vi "getGroupIdxAndLeng.vi"(8 "error in (no error)":errorcluster, 10 "DOF Group":T1, 11 "OptStateEsti in":refnum<class "OptStateEsti.lvclass">) -> (0 "error out":errorcluster, 1 "Group Length":i32, 2 "Start Index":i32, 3 "OptStateEsti out":refnum<class "OptStateEsti.lvclass">)   [LabVIEW 2016, in "OfcFunc.lvlib" / "OptStateEsti.lvclass"]
doc: "Get the start index and length of specific group of degree of freedom (DOF)."
uses:
  OptStateEsti.lvclass
  StrictDef/DofGroup.ctl
  OptStateEsti.lvclass/OptStateEsti.ctl
  <vilib>/regexp/Match Regular Expression.xnode
  MatOper/MatOper.lvclass
  OfcFunc.lvlib
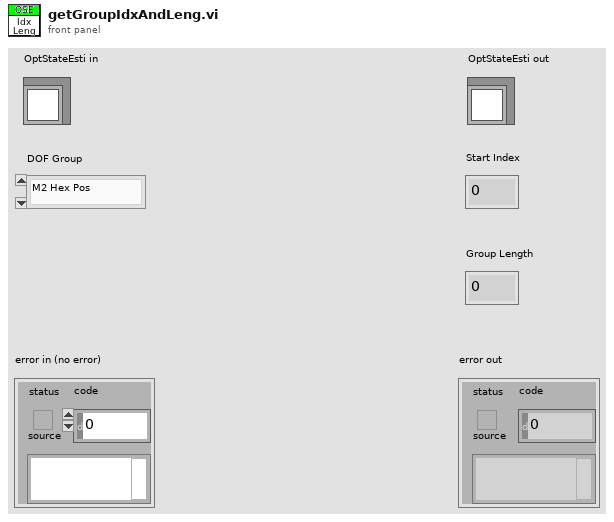
[diagram p1: front panel]
types:
  T1 = typedef "OfcFunc.lvlib/DofGroup.ctl" = enum16{"M2 Hex Pos", "Cam Hex Pos", "M1M3 Bend", "M2 Bend"}
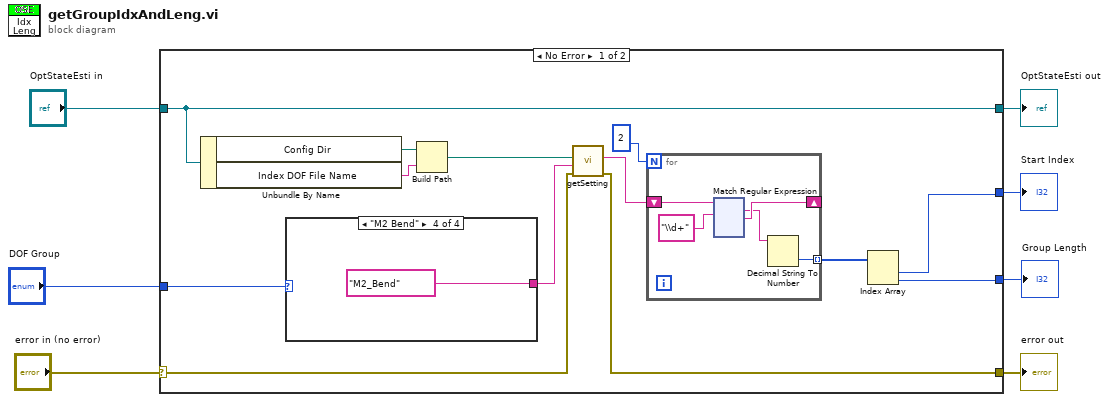
[diagram p0: block diagram]
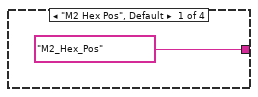
[diagram p2: hidden frame]
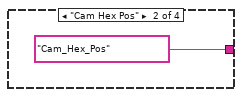
[diagram p3: hidden frame]
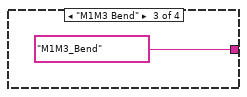
[diagram p4: hidden frame]
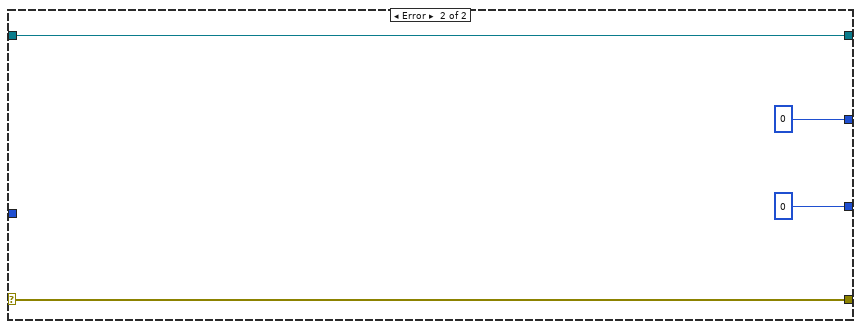
[diagram p5: hidden frame]
diagram:
  n1 = case shown="No Error" "error in (no error)" {
    selector: "error in (no error)" -> [w9 w147]
    tunnel: [w8 w147] -> w6
    tunnel: [w20 w146] -> w4
    tunnel: "OptStateEsti in" -> [w20 w146]
    tunnel: "DOF Group" -> [w18 _]
    tunnel: [w12 0] -> w2
    tunnel: [w11 0] -> w1
    frame No Error {
      n2 = Unbundle By Name(w20) -> ("Config Dir"=w19:path, "Index DOF File Name"=w10:string)
      n3 = case shown="\"M2 Bend\"" w18 {
        tunnel: ["M2_Hex_Pos" "Cam_Hex_Pos" "M1M3_Bend" "M2_Bend"] -> w16
        frame "M2 Hex Pos", Default {
        }
        frame "Cam Hex Pos" {
        }
        frame "M1M3 Bend" {
        }
        frame "M2 Bend" {
        }
      }
      n4 = Build Path(base path=w19, name or relative path=w10) -> (appended path=w17:path)
      n5 = call "getSetting.vi"("error in (no error)"=w9, "Parameter"=w16, "Path"=w17) -> ("error out"=w8:errorcluster, "Value"=w14:string)  [unwired: 6 in, 1 out]
      n6 = for {
        N: 2 -> [_]
        shift-right: [w24] -> _
        shift-left: w14 -> [w25]
        tunnel: [w21] -> w13 mode=indexing
        n7 = xnode "Match Regular Expression"("input string"=w25, "regular expression"="\\d+") -> ("whole match"=w22:string, "after match"=w24:string)  [unwired: 4 in, 3 out]
        n8 = Decimal String To Number(string=w22) -> (number=w21:i32)  [unwired: 2 in, 1 out]
      }
      n9 = Index Array(array=w13) -> (element #1=w12:i32, element #2=w11:i32)  [unwired: 2 in]
    }
    frame Error {
    }
  }
  "error out" <- w6
  "OptStateEsti out" <- w4
  "Start Index" <- w2
  "Group Length" <- w1
